vi "Read Grand Child Class Info.vi"(8 "error in (no error)":errorcluster) -> (0 "error out":errorcluster, 1 "Class Names":string[](array[string]), 2 "Library Versions":T1(array[cluster]), 3 "Private Data Clusters":variant[](array[variant]))   [LabVIEW 2017]
uses:
  GrandChildClass/GrandChildClass.lvclass
  Composition/Composition.lvlib
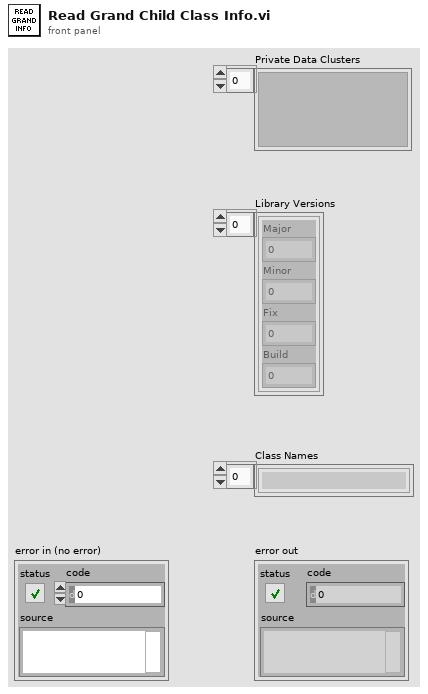
[diagram p1: front panel]
types:
  T1 = cluster{"Major":u16, "Minor":u16, "Fix":u16, "Build":u16}[]
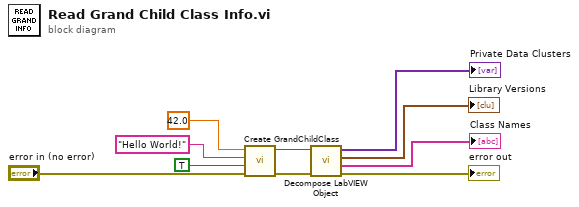
[diagram p0: block diagram]
diagram:
  n1 = call "Create GrandChildClass.vi"("error in (no error)"="error in (no error)", "Boolean"=TRUE, "String"="Hello World!", "Numeric"=42.0) -> ("error out"=w6:errorcluster, "GrandChildClass"=w4:refnum<class "GrandChildClass.lvclass">)  [unwired: 6 in]
  n2 = call "Decompose LabVIEW Object.vi"("error in (no error)"=w6, "LabVIEW Object"=w4) -> ("error out"=→"error out":errorcluster, "Class Names"=→"Class Names":string[], "Library Versions"=→"Library Versions":T1, "Private Data Clusters"=→"Private Data Clusters":variant[])  [unwired: 6 in]
